vi "CalculateHardwareData.vi"(8 "Error In":errorcluster, 11 "Hardware Collect Data":T2) -> (0 "Error Out":errorcluster, 2 "BPM":cluster{dbl[], "Beam Profile":dbl[]}[](array[cluster]), 3 "Hardware Display Data":T1)   [LabVIEW 2012]
uses:
  HardwareCollectData.ctl
  PXI6229Data.ctl
  CurrentMeterData.ctl
  HardwareDisplayData.ctl
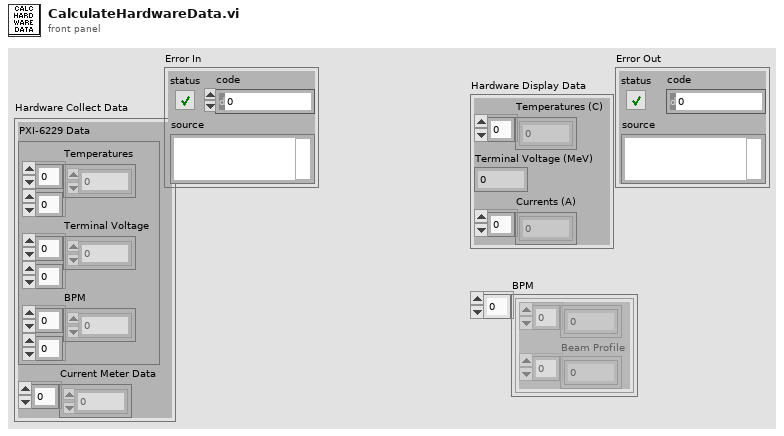
[diagram p1: front panel]
types:
  T1 = typedef "HardwareDisplayData.ctl" = cluster{"Temperatures (C)":dbl[], "Terminal Voltage (MeV)":dbl, "Currents (A)":dbl[]}
  T2 = typedef "HardwareCollectData.ctl" = cluster{"PXI-6229 Data":T3, "Current Meter Data":T4}
  T3 = typedef "PXI6229Data.ctl" = cluster{"Temperatures":dbl[][], "Terminal Voltage":dbl[][], "BPM":dbl[][]}
  T4 = typedef "CurrentMeterData.ctl" = dbl[]
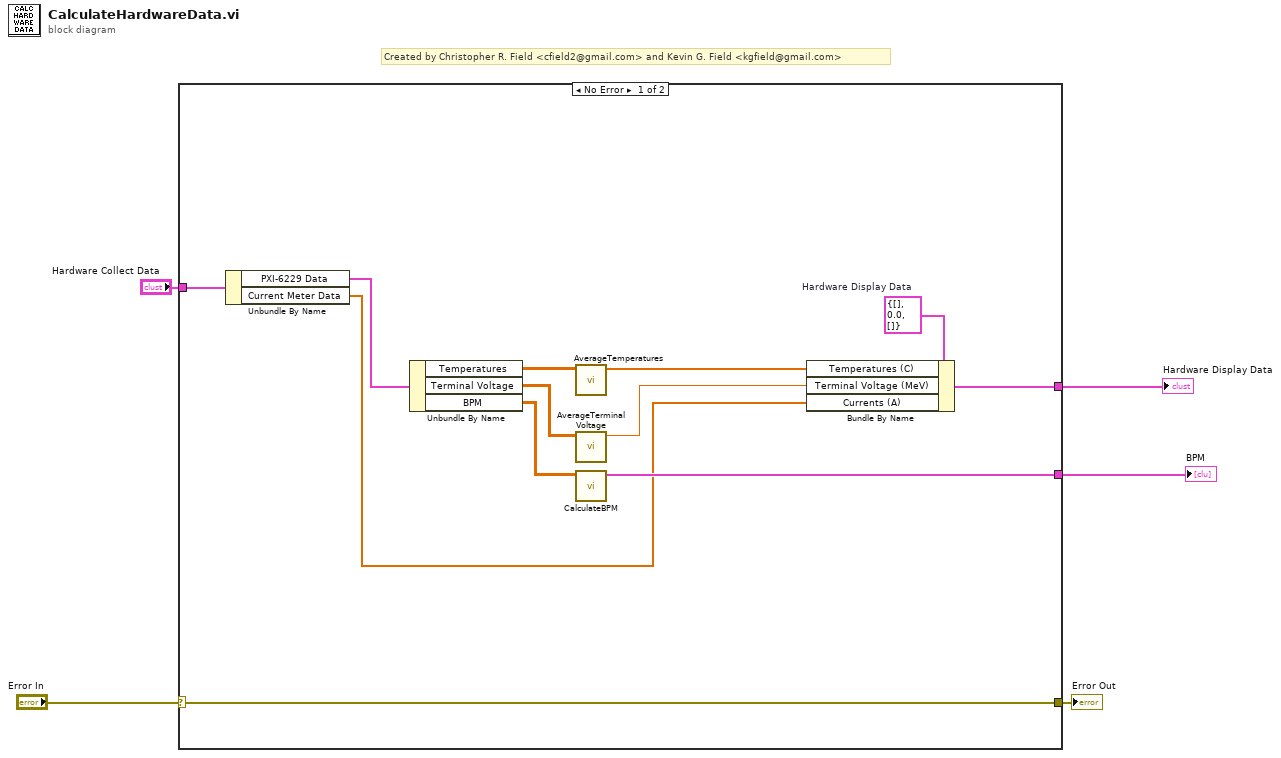
[diagram p0: block diagram]
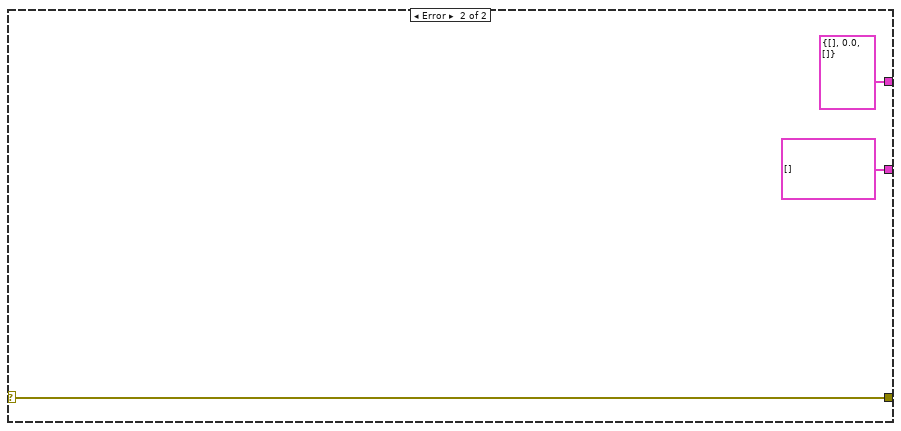
[diagram p2: hidden frame]
diagram:
  # "Created by Christopher R. Field <cfield2@gmail.com> and Kevin G. Field <kgfield@gmail.com>"
  n1 = case shown="No Error" "Error In" {
    selector: "Error In" -> [w9 w20]
    tunnel: "Hardware Collect Data" -> [w12 _]
    tunnel: [w11 T1 {"Temperatures (C)"=[], "Terminal Voltage (MeV)"=0.0, "Currents (A)"=[]} ("Hardware Display Data")] -> w4
    tunnel: [w10 cluster{dbl[], "Beam Profile":dbl[]}[] [] ("BPM")] -> w3
    tunnel: [w9 w20] -> w1
    frame No Error {
      w15 = T1 {"Temperatures (C)"=[], "Terminal Voltage (MeV)"=0.0, "Currents (A)"=[]}  # Hardware Display Data
      n2 = Unbundle By Name(w12) -> ("PXI-6229 Data"=w13:T3, "Current Meter Data"=w8:T4)
      n3 = Unbundle By Name(w13) -> ("Temperatures"=w6:dbl[][], "Terminal Voltage"=w17:dbl[][], "BPM"=w16:dbl[][])
      n4 = call "AverageTemperatures.vi"("Raw Temperatures"=w6) -> ("Temperatures (C)"=w7:dbl[])  [unwired: 10 in]
      n5 = call "AverageTerminalVoltage.vi"("Raw Terminal Voltage"=w17) -> ("Terminal Voltage (MeV)"=w14:dbl)  [unwired: 10 in]
      n6 = call "CalculateBPM.vi"("Raw Beam Profile"=w16) -> ("BPM"=w10:cluster{dbl[], "Beam Profile":dbl[]}[])  [unwired: 10 in]
      n7 = Bundle By Name(cluster=w15, "Temperatures (C)"=w7, "Terminal Voltage (MeV)"=w14, "Currents (A)"=w8) -> (w11:T1)
    }
    frame Error {
    }
  }
  "Hardware Display Data" <- w4
  "BPM" <- w3
  "Error Out" <- w1
